vi "highlightCommonEvents.vi"(8 "error in (no error)":errorcluster, 9 "Enum":enum16{"Channel Names", "Stage"}(ring), 10 "rowIndex":i32, 11 "ScriptEditorV2 in":refnum<class "ScriptEditorV2.lvclass">) -> (0 "error out":errorcluster, 3 "ScriptEditorV2 out":refnum<class "ScriptEditorV2.lvclass">)   [LabVIEW 2011, in "Views.lvlib" / "ScriptEditor.lvlib" / "ScriptEditorV2.lvclass"]
uses:
  ScriptEditorV2.lvclass
  ScriptEditorV2.lvclass/ScriptEditorV2.ctl
  Tools/Scripting/ScriptingEvent/ScriptEventList/ScriptEventList.lvclass
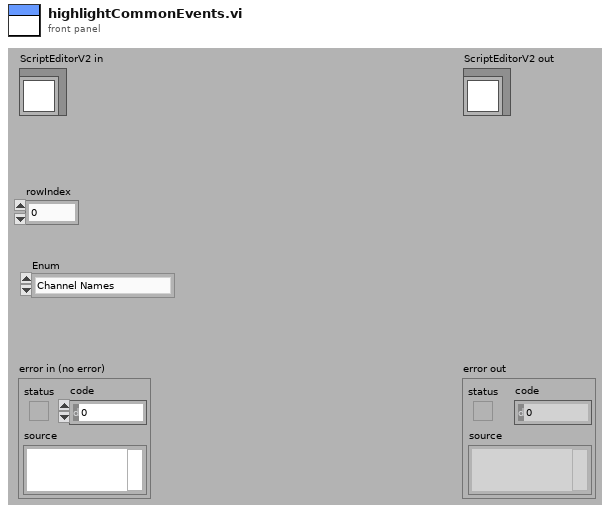
[diagram p1: front panel]
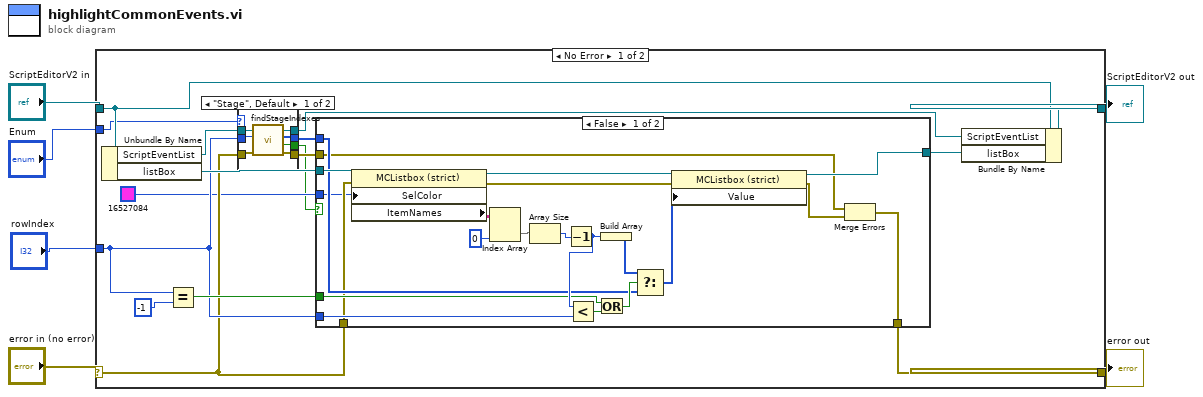
[diagram p0: block diagram]
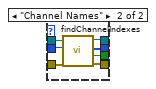
[diagram p3: hidden frame]
diagram:
  n1 = case shown="No Error" "error in (no error)" {
    selector: "error in (no error)" -> [w13 w61]
    tunnel: [w10 w61] -> w3
    tunnel: [w20 w60] -> w4
    tunnel: "ScriptEditorV2 in" -> [w21 w60]
    tunnel: "rowIndex" -> [w15 _]
    tunnel: "Enum" -> [w8 _]
    frame No Error {
      n2 = Unbundle By Name(w21) -> ("ScriptEventList"=w16:refnum<class "ScriptEventList.lvclass">, "listBox"=w22:refnum<vi>)
      n3 = Equal?(x=w15, y=-1) -> (x = y?=w17:bool)
      n4 = case shown="\"Stage\", Default" w8 {
        tunnel: w16 -> [w52 w53]
        tunnel: w15 -> [w47 w58]
        tunnel: [w50 w56] -> w14
        tunnel: w13 -> [w48 w59]
        tunnel: [w51 w57] -> w12
        tunnel: [w49 w54] -> w11
        tunnel: [w46 w55] -> w7
        frame "Stage", Default {
          n5 = call "findStageIndexes.vi"("error in (no error)"=w48, "index"=w47, "ScriptEventList in"=w52) -> ("error out"=w49:errorcluster, "noneFound"=w46:bool, "indexArray"=w50:i32[], "ScriptEventList out"=w51:refnum<class "ScriptEventList.lvclass">)  [unwired: 5 in]
        }
        frame "Channel Names" {
          n6 = call "findChannelIndexes.vi"("error in (no error)"=w59, "index"=w58, "ScriptEventList in"=w53) -> ("error out"=w54:errorcluster, "noneFound"=w55:bool, "indexArray"=w56:i32[], "ScriptEventList out"=w57:refnum<class "ScriptEventList.lvclass">)  [unwired: 5 in]
        }
      }
      n7 = case shown="False" w7 {
        tunnel: w22 -> [w43 w45]
        tunnel: [w34 w45] -> w18
        tunnel: w17 -> [w31 _]
        tunnel: w15 -> [w29 _]
        tunnel: w14 -> [w28 _]
        tunnel: w13 -> [w27 _]
        tunnel: w11 -> [w26 w44]
        tunnel: [w24 w44] -> w10
        tunnel: u32 16527084 -> [w23 _]
        frame False {
          n8 = property class="MCListbox (strict)"(reference=w43, error in=w27, "SelColor"=w23) -> (reference out=w37:refnum<vi>, error out=w35:errorcluster, "ItemNames"=w42:string[][])
          n9 = Index Array(array=w42, index (col)=0) -> (element=w40:string[])  [unwired: 1 in]
          n10 = Array Size(array=w40) -> (size(s)=w39:i32)
          n11 = Decrement(x=w39) -> (x-1=w32:i32)
          n12 = Less?(x=w32, y=w29) -> (x < y?=w33:bool)
          n13 = Or(x=w31, y=w33) -> (x .or. y?=w30:bool)
          n14 = Build Array(w32) -> (w38:i32[])
          n15 = Select(t=w38, s=w30, f=w28) -> (s? t:f=w36:i32[])
          n16 = property class="MCListbox (strict)"(reference=w37, error in=w35, "Value"=w36) -> (reference out=w34:refnum<vi>, error out=w25:errorcluster)
          n17 = Merge Errors(w26, w25) -> (w24:errorcluster)
        }
        frame True {
        }
      }
      n18 = Bundle By Name(cluster=w21, "ScriptEventList"=w12, "listBox"=w18) -> (w20:refnum<class "ScriptEditorV2.lvclass">)
    }
    frame Error {
    }
  }
  "error out" <- w3
  "ScriptEditorV2 out" <- w4
